vi "DepthSense NewFrame Callback 2.vi"(4 "User Parameter":T1, 6 "Control Ref":refnum<k24>, 7 "Event Common Data":T2) -> ()   [LabVIEW 2011]
uses:
  C:/Users/Behavior Room/Desktop/Kinect Mouse/DepthSense/FunctionPointerProxy/FunctionPointerProxy/bin/Release/FunctionPointerProxy.dll
  FunctionPointerProxy/FunctionPointerProxy/bin/Release/FunctionPointerProxy.dll
  <userlib>/libOptrima-2-3/libOptrima-2-3.lvlib
panel:
  in  "Debug?":bool
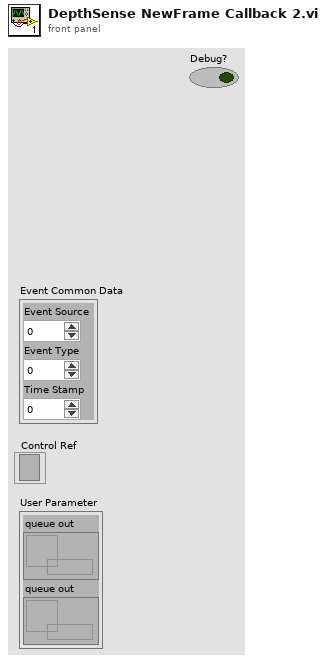
[diagram p1: front panel]
types:
  T1 = cluster{"queue out":refnum<queue>, "queue out":refnum<queue>}
  T2 = cluster{"Event Source":i32, "Event Type":u32, "Time Stamp":u32}
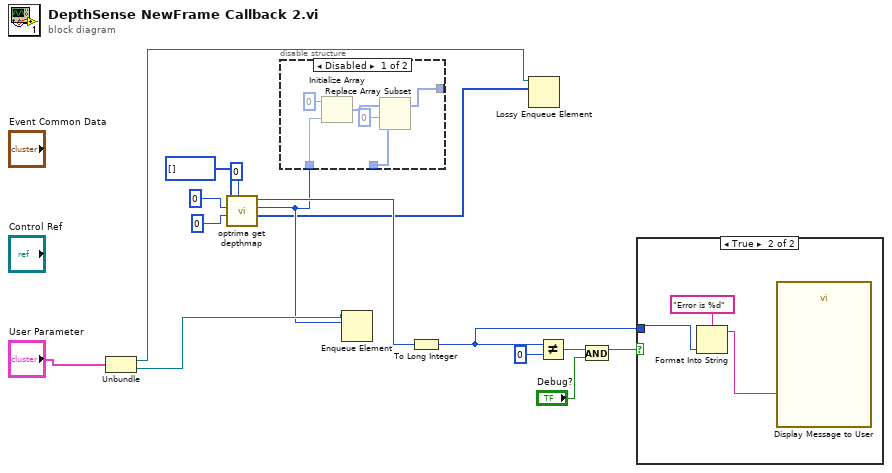
[diagram p0: block diagram]
diagram:
  n1 = Unbundle("User Parameter") -> ("queue out"=w4:refnum<queue>, "queue out"=w5:refnum<queue>)
  n2 = call <userlib>:"optrima get depthmap.vi"("to_camera_plane"=0, "confidenceTH"=i16 0 ("confidence_threshold"), "length"=u32 0, "p_depthmap in"=u16[] []) -> ("p_depthmap out"=w1:u16[], "length out"=w3:u32, "function return"=w11:u32)  [unwired: 4 in, 1 out]
  n3 = disable-structure shown="Disabled" {
    disable-tunnel: w3 -> [w21 _]
    disable-tunnel: _ -> [w17 _]
    disable-tunnel: [w16 _] -> _
    frame Disabled {
      n4 = Initialize Array(i16 0 ("element"), w21) -> (w19:i16[])
      n5 = Replace Array Subset(array=w19, new element=w17, index=0) -> (w16:i16[])
    }
    frame Enabled {
    }
  }
  n6 = Enqueue Element(queue=w5, element=w3) -> ()  [unwired: 2 in, 3 out]
  n7 = To Long Integer(number=w11) -> (32bit integer=w9:i32)
  n8 = Lossy Enqueue Element(queue=w4, element=w1) -> ()  [unwired: 1 in, 4 out]
  n9 = Not Equal?(x=w9, y=0) -> (x != y?=w7:bool)
  n10 = And(x=w7, y="Debug?") -> (x .and. y?=w8:bool)
  n11 = case shown="True" w8 {
    tunnel: w9 -> [_ w22]
    frame False {
    }
    frame True {
      n12 = Format Into String(format string="Error is %d", w22) -> (resulting string=w24:string)  [unwired: 2 in, 1 out]
      n13 = call "Display Message to User"("Message"=w24) -> ()  [unwired: 9 in, 2 out]
    }
  }
